vi "dfd_Validate Filter.vi"(8 "error in (no error)":errorcluster, 10 "check option":u16(ring) items=["Auto", "FLP Only", "FXP"], 11 "filter in":T1={"mSRate_Fs"=1.0, "mSRate_Version"="1.0", "mSRate_Comments"="", "mSRate_OrgCoef"={"type"=enum."Undefined", "gain"=1.0, "coef a (k)"=[], "coef b (v)"=[]}, "mSRate_CurCoef"={"type"=enum."Undefined", "gain"=1.0, "coef a (k)"=[], "coef b (v)"=[]}, "mSRate_Quantized?"=FALSE, "mSRate_QCoef"={"type"=enum."Undefined", "gain"=1.0, "coef a (k)"=[], "coef b (v)"=[]}, "mSRate_QSettings"=[], "mSRate_Order"=0, "mSRate_Scaling"={"mSRate_ScaleByPowerOf2?"=FALSE, "mSRate_ScaleType"=enum."No Norm"}} {"mSRate_QSettings"."source" items=["Coef a/k"=0, "Coef b/v"=7, "Input"=1, "Output"=2, "Multiplicand"=3, "Product"=4, "Sum"=5, "Delay"=6, "Gain"=8]}) -> (0 "error out":errorcluster, 2 "is Valid?":bool, 3 "filter out":T1={"mSRate_Fs"=1.0, "mSRate_Version"="1.0", "mSRate_Comments"="", "mSRate_OrgCoef"={"type"=enum."Undefined", "gain"=1.0, "coef a (k)"=[], "coef b (v)"=[]}, "mSRate_CurCoef"={"type"=enum."Undefined", "gain"=1.0, "coef a (k)"=[], "coef b (v)"=[]}, "mSRate_Quantized?"=FALSE, "mSRate_QCoef"={"type"=enum."Undefined", "gain"=1.0, "coef a (k)"=[], "coef b (v)"=[]}, "mSRate_QSettings"=[], "mSRate_Order"=0, "mSRate_Scaling"={"mSRate_ScaleByPowerOf2?"=FALSE, "mSRate_ScaleType"=enum."No Norm"}} {"mSRate_QSettings"."source" items=["Coef a/k"=0, "Coef b/v"=7, "Input"=1, "Output"=2, "Multiplicand"=3, "Product"=4, "Sum"=5, "Delay"=6, "Gain"=8]})   [LabVIEW 2017, in "NI_DigFilterLicensed.lvlib"]
uses:
  <vilib>/addons/Digital Filter Design/NI_DigFilterLicensed.lvlib
  <vilib>/addons/Digital Filter Design/_Objects.llb/DFD Filter Obj.ctl
  <vilib>/addons/Digital Filter Design/_Objects.llb/DFD Filter Coef.ctl
  <vilib>/addons/Digital Filter Design/_Objects.llb/DFD Filter Structure Type Selector.ctl
  <vilib>/addons/Digital Filter Design/_Objects.llb/dfd_Internal Quantization Settings.ctl
  <vilib>/addons/Digital Filter Design/_Objects.llb/dfd_Internal Quantization Srcs.ctl
  <vilib>/addons/Digital Filter Design/_Objects.llb/DFD Coef Norm Type.ctl
  <vilib>/addons/Digital Filter Design/_Misc.llb/dfd_Error Handlers (Single).vi
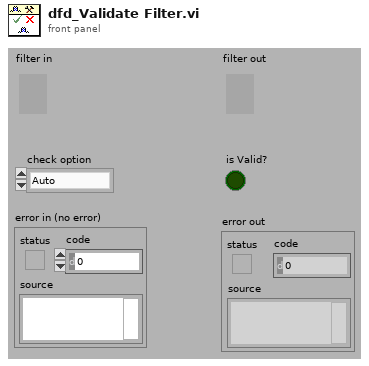
[diagram p1: front panel]
types:
  T1 = typedef "NI_DigFilterLicensed.lvlib/DFD Filter Obj.ctl" = cluster{"mSRate_Fs":dbl, "mSRate_Version":string, "mSRate_Comments":string, "mSRate_OrgCoef":T2, "mSRate_CurCoef":T2, "mSRate_Quantized?":bool, "mSRate_QCoef":T2, "mSRate_QSettings":T4[], "mSRate_Order":i32, "mSRate_Scaling":cluster{"mSRate_ScaleByPowerOf2?":bool, "mSRate_ScaleType":T6}}
  T2 = typedef "NI_DigFilterLicensed.lvlib/DFD Filter Coef.ctl" = cluster{"type":T3, "gain":dbl, "coef a (k)":dbl[], "coef b (v)":dbl[]}
  T3 = typedef "NI_DigFilterLicensed.lvlib/DFD Filter Structure Type Selector.ctl" = enum16{"Undefined", "FIR Direct Form", "FIR Direct Form Transposed", "FIR Symmetric", "FIR Antisymmetric", "IIR Direct Form I", "IIR Direct Form I Transposed", "IIR Direct Form II", "IIR Direct Form II Transposed", "IIR Cascaded Second Order Sections Form I", "IIR Cascaded Second Order Sections Form I Transposed", "IIR Cascaded Second Order Sections Form II", "IIR Cascaded Second Order Sections Form II Transposed", "Lattice Allpass (basic sections)", "Lattice Allpass (one multiplier sections)", "Lattice Allpass (normalized sections)", "Lattice AR (basic sections)", "Lattice AR (one multiplier sections)", "Lattice AR (normalized sections)", "Lattice MA (minimum phase)", "Lattice MA (maximum phase)", "Lattice ARMA (basic sections)", "Lattice ARMA (one multiplier sections)", "Lattice ARMA (normalized sections)"}
  T4 = typedef "NI_DigFilterLicensed.lvlib/dfd_Internal Quantization Settings.ctl" = cluster{"source":T5, "wl":i16, "iwl":i16, "overflow mode":enum16{"Saturation", "Wrap"}, "rounding mode":enum16{"Nearest", "Truncation"}, "signed?":bool}
  T5 = typedef "NI_DigFilterLicensed.lvlib/dfd_Internal Quantization Srcs.ctl" = u16
  T6 = typedef "NI_DigFilterLicensed.lvlib/DFD Coef Norm Type.ctl" = enum16{"No Norm", "Time Domain 1-Norm", "Time Domain 2-Norm", "Time Domain Inf-Norm"}
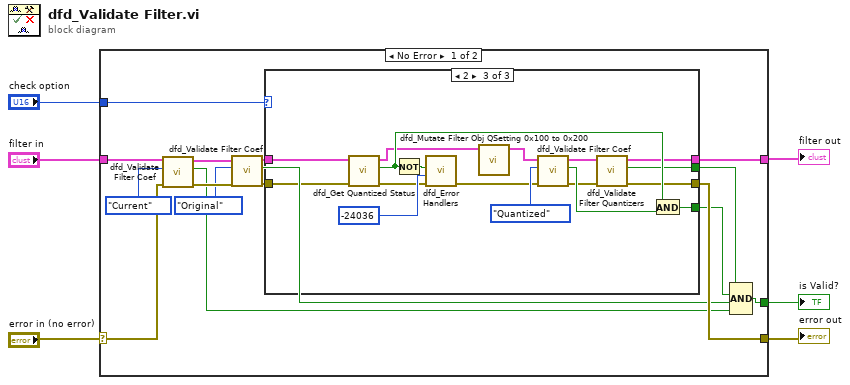
[diagram p0: block diagram]
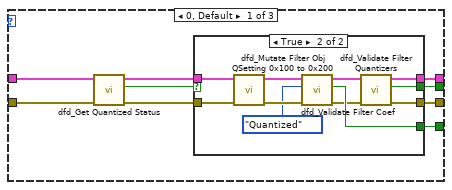
[diagram p2: hidden frame]
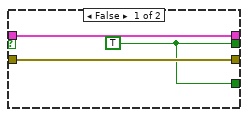
[diagram p3: hidden frame]
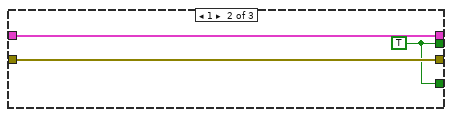
[diagram p4: hidden frame]
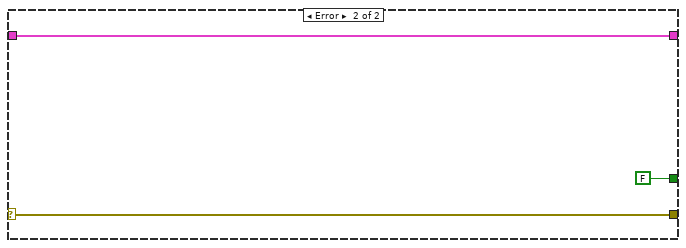
[diagram p5: hidden frame]
diagram:
  n1 = case shown="No Error" "error in (no error)" {
    selector: "error in (no error)" -> [w15 w67]
    tunnel: "filter in" -> [w20 w66]
    tunnel: [w22 w67] -> w4
    tunnel: [w21 w66] -> w3
    tunnel: [w12 FALSE] -> w2
    tunnel: "check option" -> [w8 _]
    frame No Error {
      n2 = call <vilib>:"dfd_Validate Filter Coef.vi"("error in (no error)"=w15, "coef source"=enum16{"Original", "Current", "Quantized"}."Current", "filter in"=w20) -> ("error out"=w19:errorcluster, "is Valid?"=w9:bool, "filter out"=w16:T1)  [unwired: 6 out]
      n3 = call <vilib>:"dfd_Validate Filter Coef.vi"("error in (no error)"=w19, "coef source"=enum16{"Original", "Current", "Quantized"}."Original", "filter in"=w16) -> ("error out"=w13:errorcluster, "is Valid?"=w10:bool, "filter out"=w14:T1)  [unwired: 6 out]
      n4 = case shown="2" w8 {
        tunnel: [w31 w46 w51] -> w22
        tunnel: [w30 w47 w54] -> w21
        tunnel: w14 -> [w29 w47 w64]
        tunnel: w13 -> [w28 w46 w62]
        tunnel: [w24 w45 w55] -> w11
        tunnel: [w23 w45 w53] -> w7
        frame 0, Default {
          n5 = call <vilib>:"dfd_Get Quantized Status.vi"("error in (no error)"=w28, "filter in"=w29) -> ("error out"=w26:errorcluster, "quantized?"=w25:bool, "filter out"=w27:T1)  [unwired: 7 out]
          n6 = case shown="True" w25 {
            tunnel: [w34 w38] -> w31
            tunnel: w26 -> [w34 w44]
            tunnel: w27 -> [w33 w36]
            tunnel: [w33 w40] -> w30
            tunnel: [w32 w41] -> w24
            tunnel: [w32 w37] -> w23
            frame False {
              w32 = TRUE ("is Valid?")
            }
            frame True {
              n7 = call <vilib>:"dfd_Mutate Filter Obj QSetting 0x100 to 0x200.vi"("filter in"=w36) -> ("filter out"=w35:T1)  [unwired: 10 out]
              n8 = call <vilib>:"dfd_Validate Filter Coef.vi"("error in (no error)"=w44, "coef source"=enum16{"Original", "Current", "Quantized"}."Quantized", "filter in"=w35) -> ("error out"=w39:errorcluster, "is Valid?"=w41:bool, "filter out"=w42:T1)  [unwired: 6 out]
              n9 = call <vilib>:"dfd_Validate Filter Quantizers.vi"("error in (no error)"=w39, "filter in"=w42) -> ("error out"=w38:errorcluster, "is Valid?"=w37:bool, "filter out"=w40:T1)  [unwired: 7 out]
            }
          }
        }
        frame 1 {
          w45 = TRUE ("is Valid?")
        }
        frame 2 {
          n10 = call <vilib>:"dfd_Get Quantized Status.vi"("error in (no error)"=w62, "filter in"=w64) -> ("error out"=w59:errorcluster, "quantized?"=w56:bool, "filter out"=w50:T1)  [unwired: 7 out]
          n11 = Not(x=w56) -> (.not. x?=w61:bool)
          n12 = call-poly <vilib>:"dfd_Error Handlers.vi"("error in (no error)"=w59, "error code"=-24036 ("ERR_NOT_FXP"), "condition failed?"=w61) -> ("error out"=w48:errorcluster)  [unwired: 8 out]
          n13 = call <vilib>:"dfd_Mutate Filter Obj QSetting 0x100 to 0x200.vi"("filter in"=w50) -> ("filter out"=w49:T1)  [unwired: 10 out]
          n14 = call <vilib>:"dfd_Validate Filter Coef.vi"("error in (no error)"=w48, "coef source"=enum16{"Original", "Current", "Quantized"}."Quantized", "filter in"=w49) -> ("error out"=w52:errorcluster, "is Valid?"=w57:bool, "filter out"=w63:T1)  [unwired: 6 out]
          n15 = call <vilib>:"dfd_Validate Filter Quantizers.vi"("error in (no error)"=w52, "filter in"=w63) -> ("error out"=w51:errorcluster, "is Valid?"=w53:bool, "filter out"=w54:T1)  [unwired: 7 out]
          n16 = And(x=w56, y=w57) -> (x .and. y?=w55:bool)
        }
      }
      n17 = Compound Arithmetic op=AND(w7, w11, w10, w9) -> (w12:bool)
    }
    frame Error {
    }
  }
  "filter out" <- w3
  "error out" <- w4
  "is Valid?" <- w2
